vi "Call dotNET DLL_LV2012_NI Verified.vi"() -> ()   [LabVIEW 2012]
doc: "This example VI calls the .NET DLL that accompanies it, which is a .NET class built in C# to emulate a very basic calculator."
uses:
  C:/Users/Hareth/Dropbox/Cleaning Community Examples/Mounzer/Old Examples/30-Calling dotNet assemblies in LabVIEW/TI83.dll
  TI83.dll
panel:
  out "Current Manufacturer Name":string
  out "Current Model Name":string
  in  "Manufacturer":string
  in  "Model":string
  in  "setprops":bool
  in  "getprops":bool
  out "result":dbl
  in  "divide":bool
  in  "multiply":bool
  in  "subtract":bool
  in  "add":bool
  in  "x":dbl
  in  "y":dbl
  in  "stop":bool
  # "Overview: This example VI calls the .NET DLL that accompanies it, which is a .NET class built in C# to emulate a very basic calculator.\nRequirements: LabVIEW 2012 (or compatible), .Net Framework 3.5 (or compatible) \nInstructions: \n1. Run the VI\n2. Use the buttons to get/set properties of the calculator, and to execute functions on operands x and y. \n3. Use execution highlighting to observe how the VI uses the TI83.dll to get its functionality."
  # "Invoke Methods"
  # "Operands"
  # "Operation"
  # "Result"
  # "Get/Set Properties"
  # "Values to Set"
  # "Operation"
  # "Last Read Values"
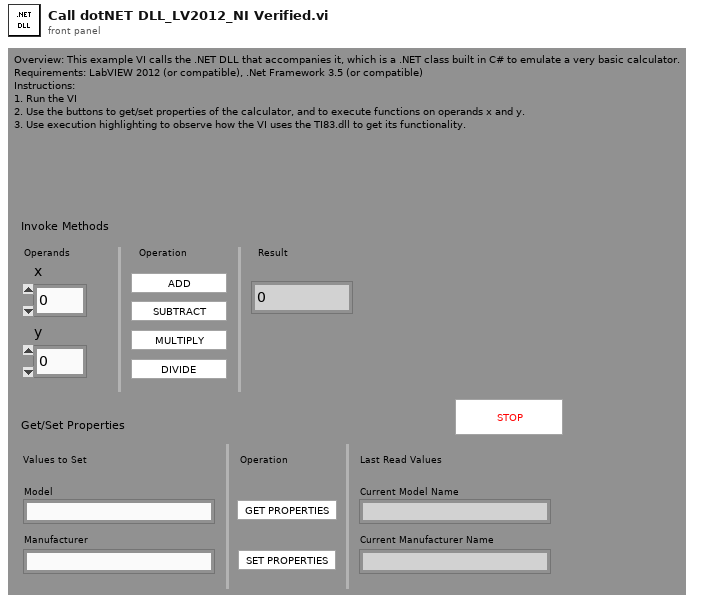
[diagram p1: front panel]
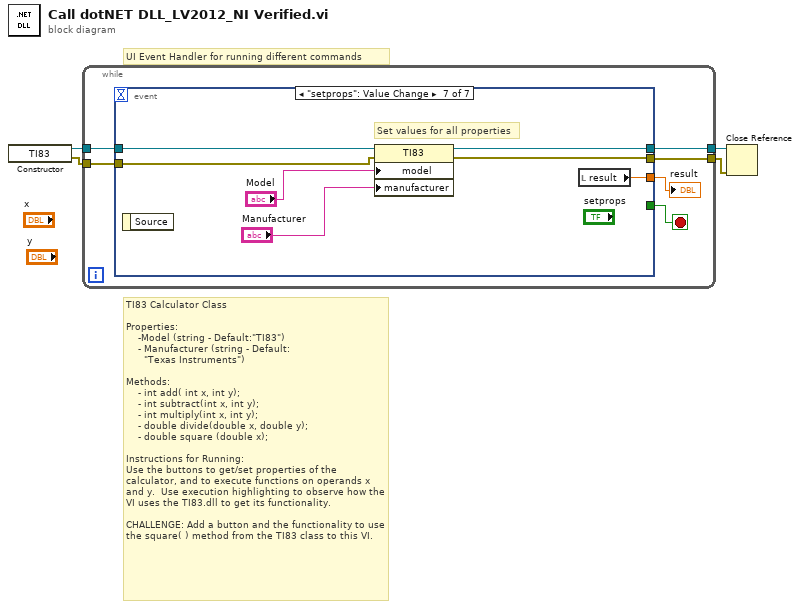
[diagram p0: block diagram]
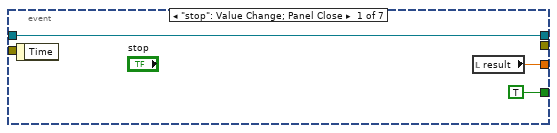
[diagram p2: hidden frame]
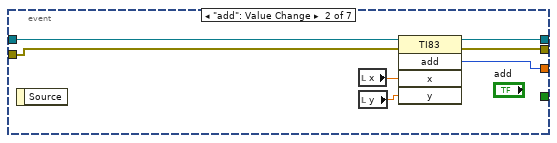
[diagram p3: hidden frame]
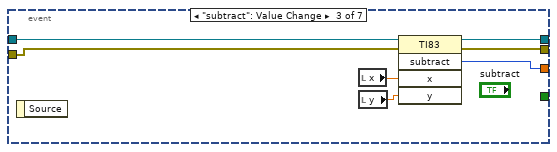
[diagram p4: hidden frame]
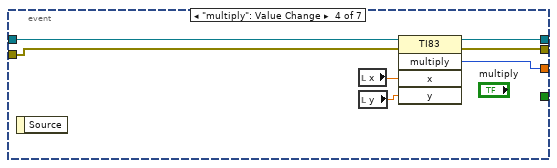
[diagram p5: hidden frame]
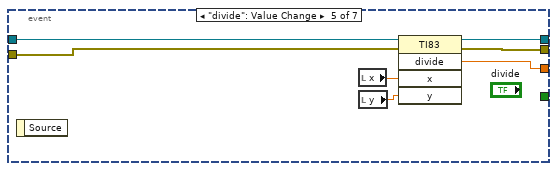
[diagram p6: hidden frame]
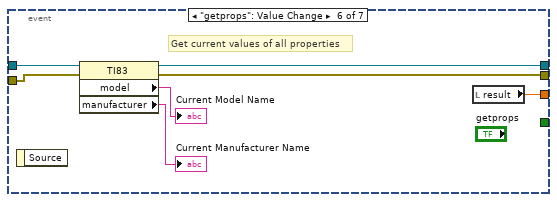
[diagram p7: hidden frame]
diagram:
  # "TI83 Calculator Class\n\nProperties:\n    -Model (string - Default:\"TI83\")\n    - Manufacturer (string - Default:\n      \"Texas Instruments\")\n\nMethods:\n    - int add( int x, int y);\n    - int subtract(int x, int y);\n    - int multiply(int x, int y);\n    - double divide(double x, double y);\n    - double square (double x);\n\nInstructions for Running:\nUse the buttons to get/set properties of the calculator, and to execute functions on operands x and y.  Use execution highlighting to observe how the VI uses the TI83.dll to get its functionality.\n\nCHALLENGE: Add a button and the functionality to use the square( ) method from the TI83 class to this VI."
  # "UI Event Handler for running different commands"
  n1 = constructor class="TI83"() -> (reference out=w4:refnum<k24>, error out=w2:errorcluster)  [unwired: 3 in, 1 out]
  n2 = while {
    tunnel: w4 -> [w9]
    tunnel: [w8] -> w3
    tunnel: w2 -> [w6]
    tunnel: [w5] -> w1
    stop <- w10 stop-if-true
    n3 = event shown="[6] \"setprops\": Value Change" {
      selector: _ -> [_ _ _ _ _ _ _]
      dyn-events: _ -> [_ _ _ _ _ _ _]
      timeout: _ -> [_ _ _ _ _ _ _]
      tunnel: [TRUE _ _ _ _ _ _] -> w10
      tunnel: w9 -> [w12 w20 w27 w34 w41 w48 w55]
      tunnel: [w12 w19 w26 w32 w40 w45 w52] -> w8
      tunnel: [w11 w18 w25 w33 w39 w44 w51] -> w7
      tunnel: w6 -> [_ w15 w22 w29 w36 w43 w50]
      tunnel: [_ w14 w21 w28 w35 w42 w49] -> w5
      event "stop": Value Change; Panel Close {
        n4 = event-data() -> ()  [unwired: 2 out]
        n5 = local read "result"() -> (w11:dbl)
      }
      event "add": Value Change {
        n6 = event-data() -> ()  [unwired: 2 out]
        n7 = local read "x"() -> (w17:dbl)
        n8 = local read "y"() -> (w16:dbl)
        n9 = invoke class="TI83" method="add"(reference=w20, error in=w15, "x"=w17, "y"=w16) -> (reference out=w19:refnum<k24>, error out=w14:errorcluster, "add"=w18:i32)  [unwired: 1 in, 2 out]
      }
      event "subtract": Value Change {
        n10 = event-data() -> ()  [unwired: 2 out]
        n11 = local read "x"() -> (w24:dbl)
        n12 = local read "y"() -> (w23:dbl)
        n13 = invoke class="TI83" method="subtract"(reference=w27, error in=w22, "x"=w24, "y"=w23) -> (reference out=w26:refnum<k24>, error out=w21:errorcluster, "subtract"=w25:i32)  [unwired: 1 in, 2 out]
      }
      event "multiply": Value Change {
        n14 = event-data() -> ()  [unwired: 2 out]
        n15 = local read "x"() -> (w31:dbl)
        n16 = local read "y"() -> (w30:dbl)
        n17 = invoke class="TI83" method="multiply"(reference=w34, error in=w29, "x"=w31, "y"=w30) -> (reference out=w32:refnum<k24>, error out=w28:errorcluster, "multiply"=w33:i32)  [unwired: 1 in, 2 out]
      }
      event "divide": Value Change {
        n18 = event-data() -> ()  [unwired: 2 out]
        n19 = local read "x"() -> (w38:dbl)
        n20 = local read "y"() -> (w37:dbl)
        n21 = invoke class="TI83" method="divide"(reference=w41, error in=w36, "x"=w38, "y"=w37) -> (reference out=w40:refnum<k24>, error out=w35:errorcluster, "divide"=w39:dbl)  [unwired: 1 in, 2 out]
      }
      event "getprops": Value Change {
        # "Get current values of all properties"
        n22 = event-data() -> ()  [unwired: 2 out]
        n23 = property class="TI83"(reference=w48, error in=w43) -> (reference out=w45:refnum<k24>, error out=w42:errorcluster, "model"=→"Current Model Name":string, "manufacturer"=→"Current Manufacturer Name":string)
        n24 = local read "result"() -> (w44:dbl)
      }
      event "setprops": Value Change {
        # "Set values for all properties"
        n25 = event-data() -> ()  [unwired: 2 out]
        n26 = property class="TI83"(reference=w55, error in=w50, "model"="Model", "manufacturer"="Manufacturer") -> (reference out=w52:refnum<k24>, error out=w49:errorcluster)
        n27 = local read "result"() -> (w51:dbl)
      }
    }
    "result" <- w7
  }
  n28 = Close Reference(reference=w3, error in (no error)=w1) -> ()  [unwired: 1 out]
